vi "Script Logging.vi"(8 "error in (no error)":errorcluster, 11 "Ballard ARINC 429 custom device in":T1 format="%.0x") -> (0 "error out":errorcluster, 2 "RT log file path":string, 3 "Ballard ARINC 429 custom device out":T1 format="%.0x")   [LabVIEW 2020]
uses:
  <vilib>/NI VeriStand/Custom Device API/Custom Device Item Ref.ctl
  Scripting/Ballard/Ballard ARINC 429 Scripting.lvlib
  <vilib>/NI VeriStand/Custom Device API/Custom Device API.lvlib
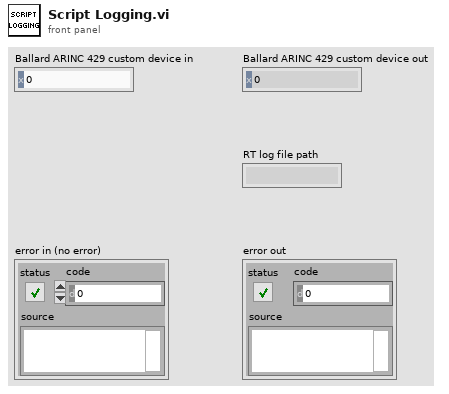
[diagram p1: front panel]
types:
  T1 = typedef "Custom Device API.lvlib/Custom Device Item Ref.ctl" = u64
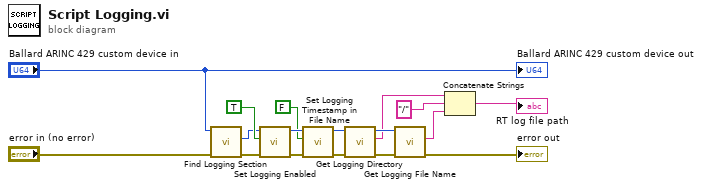
[diagram p0: block diagram]
diagram:
  n1 = call "Find Logging Section.vi"("error in"="error in (no error)", "Ballard ARINC 429 custom device in"="Ballard ARINC 429 custom device in") -> ("error out"=w5:errorcluster, "logging"=w8:T1)  [unwired: 7 in, 1 out]
  n2 = call "Set Logging Enabled.vi"("error in"=w5, "logging enabled"=TRUE, "logging in"=w8) -> ("error out"=w12:errorcluster, "logging out"=w13:T1)  [unwired: 7 in]
  n3 = call "Set Logging Timestamp in File Name.vi"("error in"=w12, "timestamp in file name"=FALSE, "logging in"=w13) -> ("error out"=w10:errorcluster, "logging out"=w16:T1)  [unwired: 7 in]
  n4 = call "Get Logging Directory.vi"("error in"=w10, "logging in"=w16) -> ("error out"=w15:errorcluster, "directory"=w3:string, "logging out"=w17:T1)  [unwired: 7 in]
  n5 = call "Get Logging File Name.vi"("error in"=w15, "logging in"=w17) -> ("error out"=→"error out":errorcluster, "file name"=w4:string)  [unwired: 7 in, 1 out]
  n6 = Concatenate Strings(w3, "/" ("string"), w4) -> (→"RT log file path":string)
  "Ballard ARINC 429 custom device out" <- "Ballard ARINC 429 custom device in"
